vi "4 Ch Digital Input.vi"(2 "4 Ch Digital In":T1={"DI0"="Chassis1/Mod4/DI0", "DI1"="Chassis1/Mod4/DI0", "DI2"="Chassis1/Mod4/DI0", "DI3"="Chassis1/Mod4/DI0"}) -> (7 "Packet":u64)   [LabVIEW 2010]
uses:
  <vilib>/eio/EIONode/EIONode.xnode
  <vilib>/rvi/eio/nirviEIOImplementation/nirviEIOImplementation.xnode
  <vilib>/rvi/eio/common/nirviEmuClasses.ctl
  <vilib>/rvi/eio/common/nirviEmuTemplateMethod_noerrors.vi
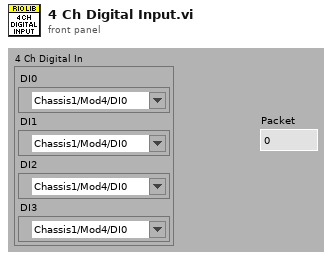
[diagram p1: front panel]
types:
  T1 = cluster{"DI0":refnum<k21>, "DI1":refnum<k21>, "DI2":refnum<k21>, "DI3":refnum<k21>}
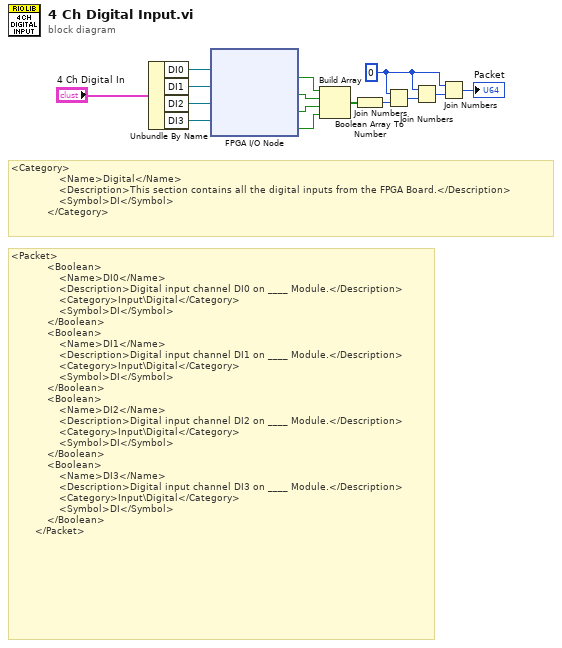
[diagram p0: block diagram]
diagram:
  w1 = u8 0 ("hi")
  # "<Category>\n                <Name>Digital</Name>\n                <Description>This section contains all the digital inputs from the FPGA Board.</Description>\n                <Symbol>DI</Symbol>\n            </Category>"
  # "<Packet>\n            <Boolean>\n                <Name>DI0</Name>\n                <Description>Digital input channel DI0 on ____ Module.</Description>\n                <Category>Input\\Digital</Category>\n                <Symbol>DI</Symbol>\n            </Boolean>\n            <Boolean>\n                <Name>DI1</Name>\n                <Description>Digital input channel DI1 on ____ Module.</Description>\n                <Category>Input\\Digital</Category>\n                <Symbol>DI</Symbol>\n            </Boolean>\n            <Boolean>\n                <Name>DI2</Name>\n                <Description>Digital input channel DI2 on ____ Module.</Description>\n                <Category>Input\\Digital</Category>\n                <Symbol>DI</Symbol>\n            </Boolean>\n            <Boolean>\n                <Name>DI3</Name>\n                <Description>Digital input channel DI3 on ____ Module.</Description>\n                <Category>Input\\Digital</Category>\n                <Symbol>DI</Symbol>\n            </Boolean>\n        </Packet>"
  n1 = Unbundle By Name("4 Ch Digital In") -> ("DI0"=w12:refnum<k21>, "DI1"=w15:refnum<k21>, "DI2"=w14:refnum<k21>, "DI3"=w13:refnum<k21>)
  n2 = xnode "FPGA I/O Node"("FPGA I/O In"=w12, "FPGA I/O In"=w15, "FPGA I/O In"=w14, "FPGA I/O In"=w13) -> ("I/O Item"=w7:bool, "I/O Item"=w9:bool, "I/O Item"=w10:bool, "I/O Item"=w8:bool)  [unwired: 4 out]
  n3 = Build Array(w7, w9, w10, w8) -> (w6:bool[])
  n4 = Boolean Array To Number(Boolean array=w6) -> (number=w5:u8)
  n5 = Join Numbers(hi=w1, lo=w5) -> ((hi.lo)=w4:u16)
  n6 = Join Numbers(hi=w1, lo=w4) -> ((hi.lo)=w3:u32)
  n7 = Join Numbers(hi=w1, lo=w3) -> ((hi.lo)=→"Packet":u64)
